vi "Offset.vi"(1 "Number":dbl) -> (0 "Ofsetted Number":dbl)   [LabVIEW 2014]
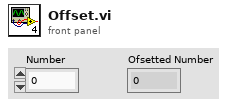
[diagram p1: front panel]
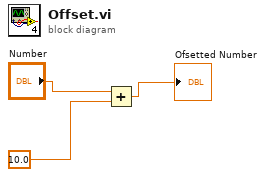
[diagram p0: block diagram]
diagram:
  n1 = Add(x="Number", y=10.0) -> (x+y=→"Ofsetted Number":dbl)
